vi "Change DocumentPath.vi"(8 "error in (no error)":errorcluster, 9 "Copy CHM path":bool, 10 "Help.Path":path, 11 "Help:Document Path W":refnum<vi>) -> (0 "error out":errorcluster)   [LabVIEW 2020]
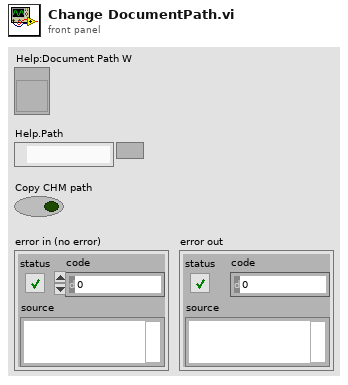
[diagram p1: front panel]
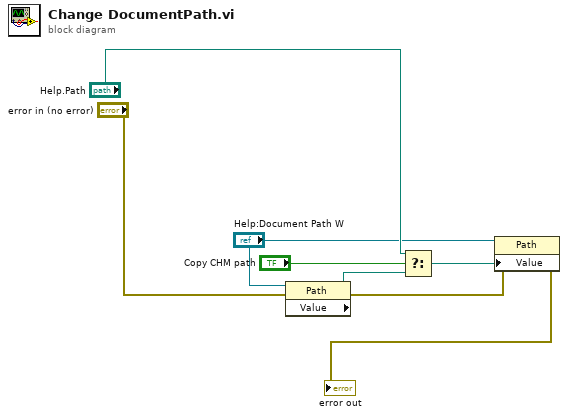
[diagram p0: block diagram]
diagram:
  n1 = property on="Property Node" class="Path"(reference="Help:Document Path W", error in="error in (no error)") -> (error out=w7:errorcluster, "Value"=w5:path)  [unwired: 1 out]
  n2 = Select(t="Help.Path", s="Copy CHM path", f=w5) -> (s? t:f=w4:path)
  n3 = property on="Property Node" class="Path"(reference="Help:Document Path W", error in=w7, "Value"=w4) -> (error out=→"error out":errorcluster)  [unwired: 1 out]
